vi "Write Com port Name.vi"(10 "Com port Name":string, 11 "Device in":refnum<class "PIC-Device.lvclass">) -> (3 "Device out":refnum<class "PIC-Device.lvclass">)   [LabVIEW 2020, in "PIC-Device.lvclass"]
uses:
  PIC-Device.lvclass
  PIC-Device.lvclass/PIC-Device.ctl
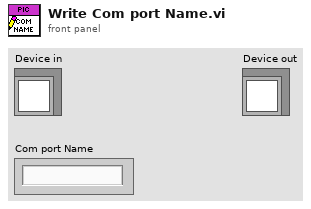
[diagram p1: front panel]
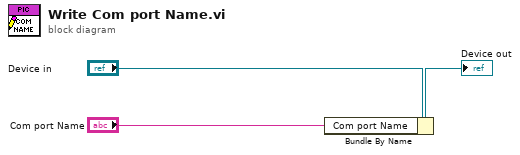
[diagram p0: block diagram]
diagram:
  n1 = Bundle By Name(cluster="Device in", "Com port Name"="Com port Name") -> (→"Device out":refnum<class "PIC-Device.lvclass">)
